vi "Get Linear Position Delta Using Encoders.vi"() -> (3 "Change in Linear Position (mm)":dbl)   [LabVIEW 2017]
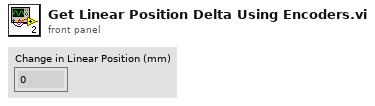
[diagram p1: front panel]
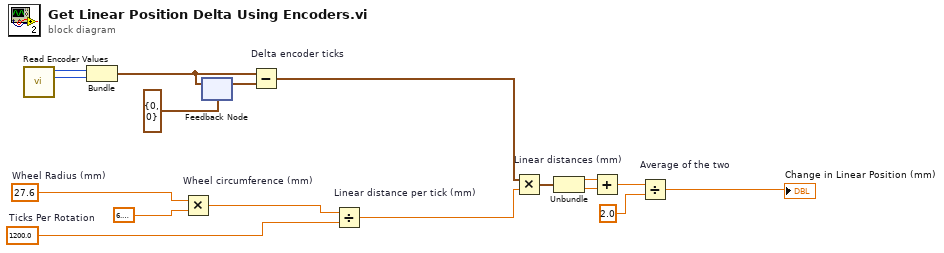
[diagram p0: block diagram]
diagram:
  w15 = 1200.0  # Ticks Per Rotation
  w5 = 27.6  # Wheel Radius (mm)
  n1 = call "Read Encoder Values.vi"() -> ("Right Value"=w17:i32, "Left  Value"=w16:i32)  [unwired: 10 in]
  n2 = Bundle("Left  Value"=w16, "Right Value"=w17) -> (w14:cluster{"Left  Value":i32, "Right Value":i32})  [unwired: 1 in]
  n3 = Multiply "Wheel circumference (mm)"(x=w5, y=6.283185307179586) -> (x*y=w4:dbl)
  n4 = feedback #1(cluster{"Left  Value":i32, "Right Value":i32} {"Left  Value"=0, "Right Value"=0}) -> (w13:cluster{"Left  Value":i32, "Right Value":i32})
  n5 = feedback-in #1(w14) -> ()
  n6 = Subtract "Delta encoder ticks"(x=w14, y=w13) -> (x-y=w2:cluster{"Left  Value":i32, "Right Value":i32})
  n7 = Divide "Linear distance per tick (mm)"(x=w4, y=w15) -> (x/y=w3:dbl)
  n8 = Multiply "Linear distances (mm)"(x=w2, y=w3) -> (x*y=w9:cluster{"Left  Value":dbl, "Right Value":dbl})
  n9 = Unbundle(w9) -> ("Left  Value"=w10:dbl, "Right Value"=w11:dbl)
  n10 = Add(x=w10, y=w11) -> (x+y=w8:dbl)
  n11 = Divide "Average of the two"(x=w8, y=2.0) -> (x/y=→"Change in Linear Position (mm)":dbl)
